vi "MathCad_App_Close.vi"(8 "error in (no error)":errorcluster, 10 "Hide Only (don't Close)":bool, 11 "Mathcad Application Reference":refnum<k7>) -> (0 "error out (no error)":errorcluster)   [LabVIEW 2015]
doc: "Closes a Mathcad Application.\n\nInputs\nMathcad Application Reference - Reference to MathcadA pplication Class that is to be closed. (All open subclass references should be closed before the IMathcadApplication Class reference is closed)\n\nOutputs\n(Error Out only)"
panel:
  in  "SaveOption":i32(ring)=2 items=["mcSaveChanges", "mcPromptToSaveChanges", "mcDiscardChanges"]
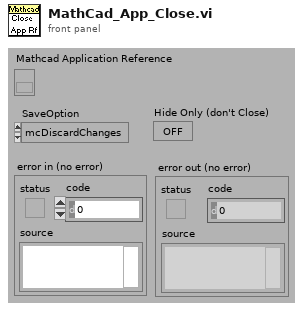
[diagram p1: front panel]
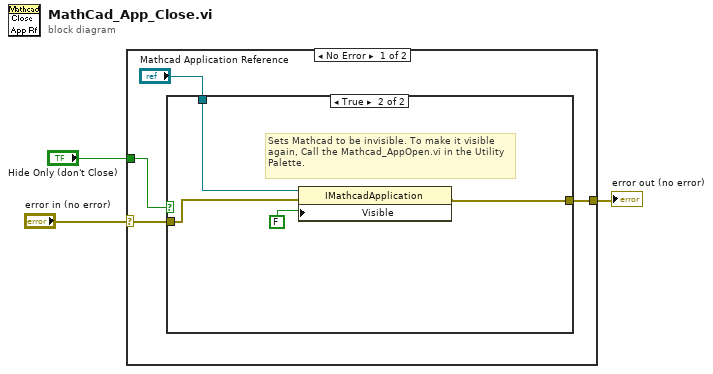
[diagram p0: block diagram]
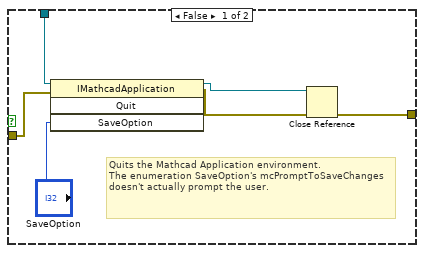
[diagram p2: hidden frame]
diagram:
  n1 = case shown="No Error" "error in (no error)" {
    selector: "error in (no error)" -> [w4 w18]
    tunnel: [w7 w18] -> w3
    tunnel: "Hide Only (don't Close)" -> [w5 _]
    frame No Error {
      n2 = case shown="True" w5 {
        tunnel: [w13 w15] -> w7
        tunnel: "Mathcad Application Reference" -> [w9 w17]
        tunnel: w4 -> [w8 w14]
        frame False {
          # "Quits the Mathcad Application environment.\nThe enumeration SaveOption's mcPromptToSaveChanges doesn't actually prompt the user."
          n3 = invoke class="IMathcadApplication" method="Quit"(reference=w9, error in=w8, "SaveOption"="SaveOption") -> (reference out=w10:refnum<k7>, error out=w11:errorcluster)  [unwired: 1 in, 2 out]
          n4 = Close Reference(reference=w10, error in (no error)=w11) -> (error out=w13:errorcluster)
        }
        frame True {
          # "Sets Mathcad to be invisible. To make it visible again, Call the Mathcad_AppOpen.vi in the Utility Palette."
          n5 = property class="IMathcadApplication"(reference=w17, error in=w14, "Visible"=FALSE) -> (error out=w15:errorcluster)  [unwired: 1 out]
        }
      }
    }
    frame Error {
    }
  }
  "error out (no error)" <- w3
